vi "Simple cDAQ thermocouple example.vi"() -> ()   [LabVIEW 2015]
panel:
  out "Temperature":dbl(graph)
  out "Loop counter":i32
  in  "stop":bool
  out "Temperature":dbl
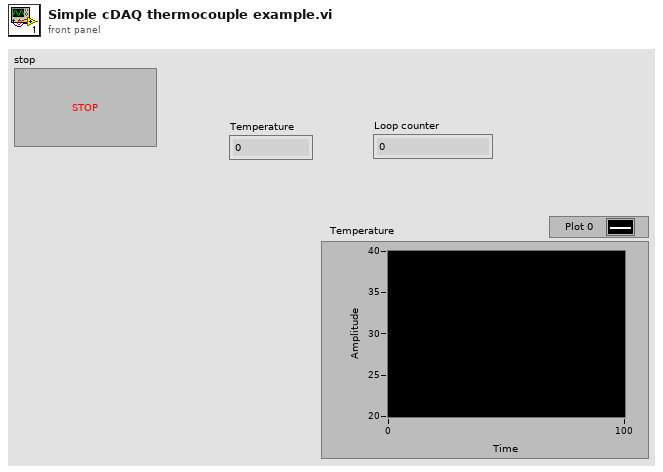
[diagram p1: front panel]
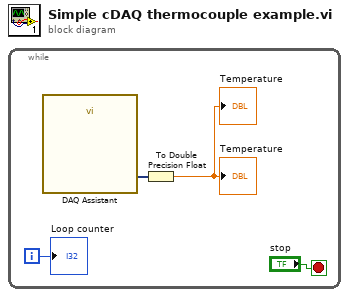
[diagram p0: block diagram]
diagram:
  n1 = while {
    i -> [w3]
    stop <- "stop" stop-if-true
    n2 = call "DAQ Assistant"() -> ("data"=w1:dynamicdata)  [unwired: 16 in, 3 out]
    n3 = To Double Precision Float(number=w1) -> (double precision float=→"Temperature" →"Temperature":dbl)
    "Loop counter" <- w3
  }
